vi "hahahhaha1.vi"() -> ()   [LabVIEW 2020]
panel:
  in  "input x2":dbl
  out "output x1+x2":dbl
  in  "input x1":dbl
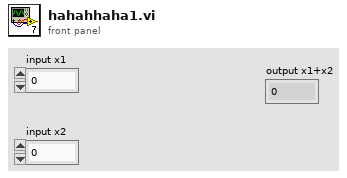
[diagram p1: front panel]
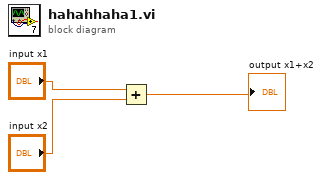
[diagram p0: block diagram]
diagram:
  n1 = Add(x="input x1", y="input x2") -> (x+y=→"output x1+x2":dbl)
